vi "SSVectorLagrange.vi"() -> (0 "D":dbl[][](array[numeric]), 1 "C":dbl[][](array[numeric]), 2 "B":dbl[][](array[numeric]), 3 "A":dbl[][](array[numeric]))   [LabVIEW 2012]
uses:
  <vilib>/imath/engines/lvmath2/RunTimeEngine/ErrorHandling/NIMS_Finalize Error.vi
  <vilib>/imath/engines/lvmath2/RunTimeEngine/Managers/WorkSpace/UID Generator.vi
  <vilib>/imath/engines/lvmath2/RunTimeEngine/Managers/SymbolTable/Clear UID.vi
  <vilib>/imath/engines/lvmath2/RunTimeEngine/NodeEndStatement/NIMS_NodeEndStatement_Output.vi
  <instcachedir>/0/NIMS_NodeEndStatement_Output_53EC0D466D134D7ABD903AC30B43404B.lvgen/NIMS_NodeEndStatement_Output_53EC0D466D134D7ABD903AC30B43404B_002.vi
  <vilib>/imath/engines/lvmath2/RunTimeEngine/ReplaceToken/NIMS_Replace - Check Row.vi
  <instcachedir>/0/NIMS_Replace - Check Row_8C35B66FE73A429EAC382AAA935851F0.lvgen/NIMS_Replace - Check Row_8C35B66FE73A429EAC382AAA935851F0_000.vi
  <vilib>/imath/engines/lvmath2/RunTimeEngine/ReplaceToken/NIMS_Replace - Check Column.vi
  <instcachedir>/0/NIMS_Replace - Check Column_F9ADE87E459D46779ACFAE3AFB317B9B.lvgen/NIMS_Replace - Check Column_F9ADE87E459D46779ACFAE3AFB317B9B_001.vi
  <vilib>/imath/engines/lvmath2/RunTimeEngine/ReplaceToken/NIMS_Replace - Size Check M(_,_)=S.vi
  <instcachedir>/0/NIMS_Replace - Size Check M(_,_)=S_0CFA00F12BB840EDA61E43D782562782.lvgen/NIMS_Replace - Size Check M(_,_)=S_0CFA00F12BB840EDA61E43D782562782_000.vi
  <vilib>/imath/engines/lvmath2/RunTimeEngine/ReplaceToken/NIMS_Replace - M(S,S)=S.vi
  <instcachedir>/0/NIMS_Replace - M(S,S)=S_59120E3D3E804D63A1B2B7FDD4B95F55.lvgen/NIMS_Replace - M(S,S)=S_59120E3D3E804D63A1B2B7FDD4B95F55_000.vi
  <vilib>/imathl/engines/lvmath/Functions/Error Handling/Create Error.vi
  <vilib>/imath/engines/lvmath2/RunTimeEngine/RunTimeType/NIMS_RunTimeType_From StrictType (excl LVString).vi
  <instcachedir>/0/NIMS_RunTimeType_From StrictType (excl LVString)_AC52D965D0864706932D20A05968E122.lvgen/NIMS_RunTimeType_From StrictType (excl LVString)_AC52D965D0864706932D20A05968E122_000.vi
  <vilib>/imath/engines/lvmath2/RunTimeEngine/LocalVariableDefStatement/MC_LocalVariableDefStatement_Display.vi
  <instcachedir>/0/NIMS_Replace - Check Row_8C35B66FE73A429EAC382AAA935851F0.lvgen/NIMS_Replace - Check Row_8C35B66FE73A429EAC382AAA935851F0_005.vi
  <instcachedir>/0/NIMS_Replace - Check Column_F9ADE87E459D46779ACFAE3AFB317B9B.lvgen/NIMS_Replace - Check Column_F9ADE87E459D46779ACFAE3AFB317B9B_007.vi
  <instcachedir>/0/NIMS_Replace - Size Check M(_,_)=S_0CFA00F12BB840EDA61E43D782562782.lvgen/NIMS_Replace - Size Check M(_,_)=S_0CFA00F12BB840EDA61E43D782562782_002.vi
  <instcachedir>/0/NIMS_Replace - M(S,S)=S_59120E3D3E804D63A1B2B7FDD4B95F55.lvgen/NIMS_Replace - M(S,S)=S_59120E3D3E804D63A1B2B7FDD4B95F55_002.vi
  <vilib>/imath/engines/lvmath2/RunTimeEngine/Managers/SymbolTable/NIMS_WorkSpace.lvlib
panel:
  in  "Moment of Inetia of the frame wrt to center of mass (Ifg)":dbl=20.0
  in  "Distance from center of wheel to center of mass (Rf)":dbl=0.463
  in  "Radius of Wheel (Rw)":dbl=0.2032
  in  "Moment of Inertia wrt center of mass (Iwg)":dbl=0.0812
  in  "Mass of Frame (mf)":dbl=25.0
  in  "Mass of Bottom Wheel (mw)":dbl=7.645
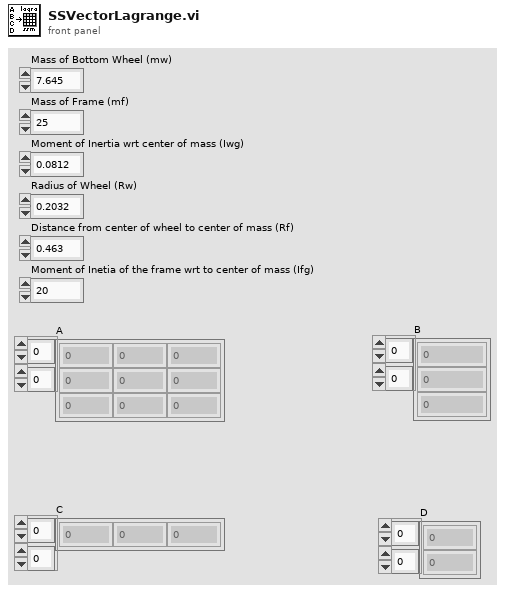
[diagram p1: front panel]
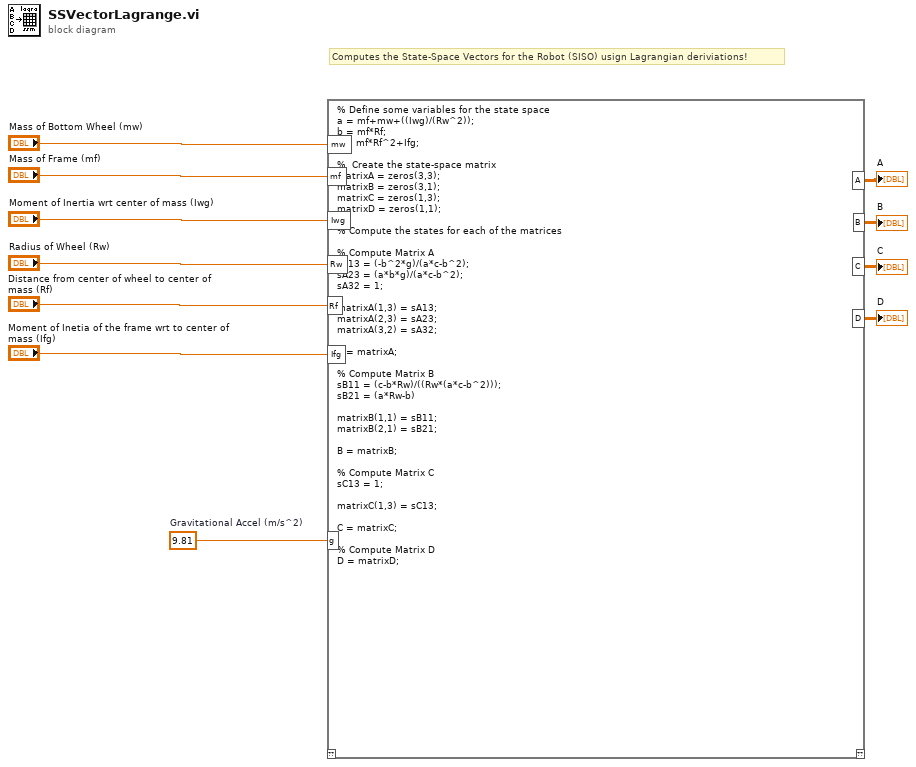
[diagram p0: block diagram]
diagram:
  w9 = 9.81  # Gravitational Accel (m/s^2)
  # "Computes the State-Space Vectors for the Robot (SISO) usign Lagrangian deriviations!"
  n1 = mathscript code="% Define some variables for the state space\na = mf+mw+((Iwg)/(Rw^2));\nb = mf*Rf;\nc = mf*Rf^2+Ifg;\n\n%  Create the state-space matrix\nmatrixA = zeros(3,3);\nmatrixB = zeros(3,1);\nmatrixC = zeros(1,3);\nmatrixD = zeros(1,1);\n\n% Compute the states for each of the matrices\n\n% Compute Matrix A\nsA13 = (-b^2*g)/(a*c-b^2);\nsA23 = (a*b*g)/(a*c-b^2);\nsA32 = 1;\n\nmatrixA(1,3) = sA13;\nmatrixA(2,3) = sA23;\nmatrixA(3,2) = sA32;\n\nA = matrixA;\n\n% Compute Matrix B\nsB11 = (c-b*Rw)/((Rw*(a*c-b^2)));\nsB21 = (a*Rw-b)\n\nmatrixB(1,1) = sB11;\nmatrixB(2,1) = sB21;\n\nB = matrixB;\n\n% Compute Matrix C\nsC13 = 1;\n\nmatrixC(1,3) = sC13;\n\nC = matrixC;\n\n% Compute Matrix D\nD = matrixD;"("mw"="Mass of Bottom Wheel (mw)", "mf"="Mass of Frame (mf)", "g"=w9, "Iwg"="Moment of Inertia wrt center of mass (Iwg)", "Rw"="Radius of Wheel (Rw)", "Rf"="Distance from center of wheel to center of mass (Rf)", "Ifg"="Moment of Inetia of the frame wrt to center of mass (Ifg)") -> ("A"=→"A":dbl[][], "B"=→"B":dbl[][], "C"=→"C":dbl[][], "D"=→"D":dbl[][])  [unwired: 1 in, 1 out]
